vi "ObstacleOurRadius.vi"(8 "Goal":dbl[](array[numeric]), 9 "Initial State":dbl[](array[numeric]), 10 "other robot":T1={"id"=0, "function"=enum."Attacker", "x"=0.0, "y"=0.0, "orientation"=0.0, "v_tangent"=0.0, "v_normal"=0.0, "v_ang"=0.0, "kick_x"=0.0, "kick_z"=0.0, "dribble"=FALSE, "Timestamp"=timestamp(0 s since 1904-01-01), "estimatives"={"est_v_tangent"=0.0, "est_v_normal"=0.0, "est_vx"=0.0, "est_vy"=0.0, "Pos Robot Est"=[]}, "dest_x_kick"=0.0, "dest_y_kick"=0.0, "Gap Coord"=[], "States"=enum."GoToTangent", "Path "=[], "Path  Smooth"=[], "Dest"=[]}) -> (2 "obstacle enemy radius":dbl)   [LabVIEW 2017]
uses:
  Core/AI Robot.ctl
  Intel/Functions Enum.ctl
  Intel/AttackerStates.ctl
  PathDests.ctl
  PathDest.ctl
  <vilib>/Analysis/_algsub.llb/Real Vector Norm.vi
  <vilib>/Analysis/NI_AALPro.lvlib
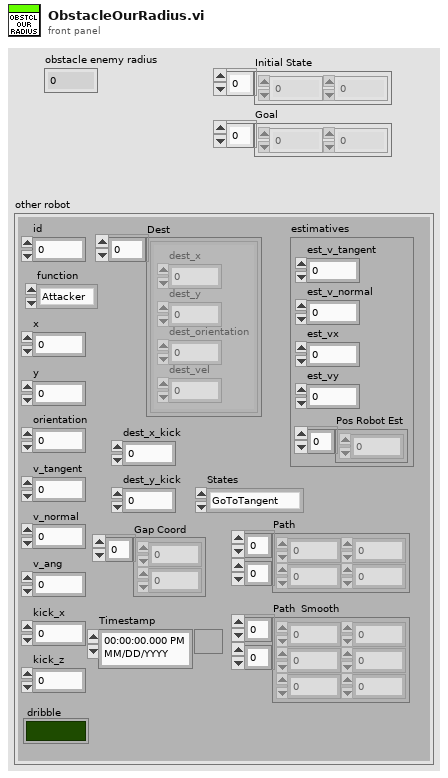
[diagram p1: front panel]
types:
  T1 = typedef "AI Robot.ctl" = cluster{"id":u32, "function":T2, "x":dbl, "y":dbl, "orientation":dbl, "v_tangent":dbl, "v_normal":dbl, "v_ang":dbl, "kick_x":dbl, "kick_z":dbl, "dribble":bool, "Timestamp":timestamp, "estimatives":cluster{"est_v_tangent":dbl, "est_v_normal":dbl, "est_vx":dbl, "est_vy":dbl, "Pos Robot Est":dbl[]}, "dest_x_kick":dbl, "dest_y_kick":dbl, "Gap Coord":dbl[], "States":T3, "Path ":dbl[][], "Path  Smooth":dbl[][], "Dest":T4}
  T2 = typedef "Functions Enum.ctl" = enum16{"Attacker", "Goalie", "Defender", "Striker", "Goto 0", "Dummy", "Kicker", "ZigZag"}
  T3 = typedef "AttackerStates.ctl" = enum16{"Pass", "GoToTangent", "BallGetting", "GoToKick", ""}
  T4 = typedef "PathDests.ctl" = T5[]
  T5 = typedef "PathDest.ctl" = cluster{"dest_x":dbl, "dest_y":dbl, "dest_orientation":dbl, "dest_vel":dbl}
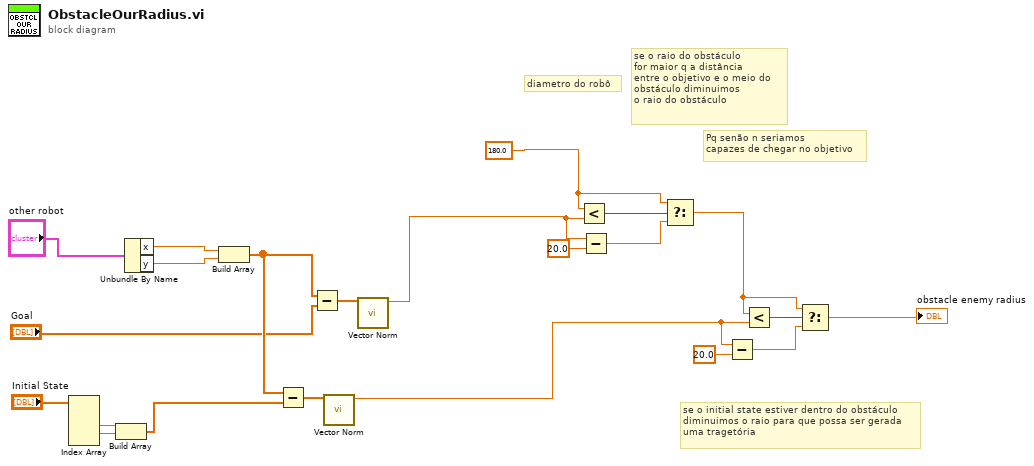
[diagram p0: block diagram]
diagram:
  w1 = 180.0 ("x")
  # "se o initial state estiver dentro do obstáculo\ndiminuimos o raio para que possa ser gerada\numa tragetória"
  # "diametro do robô"
  # "Pq senão n seriamos\ncapazes de chegar no objetivo"
  # "se o raio do obstáculo\nfor maior q a distância \nentre o objetivo e o meio do \nobstáculo diminuimos \no raio do obstáculo"
  n1 = Index Array(array="Initial State") -> (element #2=w4:dbl, element #3=w3:dbl)  [unwired: 4 in, 2 out]
  n2 = Build Array(w4, w3) -> (w2:dbl[])
  n3 = Unbundle By Name("other robot") -> ("x"=w21:dbl, "y"=w20:dbl)
  n4 = Build Array(w21, w20) -> (w13:dbl[])
  n5 = Subtract(x=w13, y=w2) -> (x-y=w14:dbl[])
  n6 = Subtract(x=w13, y="Goal") -> (x-y=w19:dbl[])
  n7 = call-poly <vilib>:"Vector Norm.vi"("Input Vector"=w14) -> ("norm"=w7:dbl)  [unwired: 9 in, 1 out]
  n8 = call-poly <vilib>:"Vector Norm.vi"("Input Vector"=w19) -> ("norm"=w17:dbl)  [unwired: 9 in, 1 out]
  n9 = Less?(x=w1, y=w17) -> (x < y?=w18:bool)
  n10 = Subtract(x=w17, y=20.0) -> (x-y=w15:dbl)
  n11 = Select(t=w1, s=w18, f=w15) -> (s? t:f=w9:dbl)
  n12 = Subtract(x=w7, y=20.0) -> (x-y=w6:dbl)
  n13 = Less?(x=w9, y=w7) -> (x < y?=w11:bool)
  n14 = Select(t=w9, s=w11, f=w6) -> (s? t:f=→"obstacle enemy radius":dbl)
